vi "Odour_stim_valve_waveforms.vi"(1 "Odour bottles":T1(array[cluster])=[[{"Mixture components"=[{"Name"="MINERAL OIL", "CID"=0, "Volatility"=0.0}], "Name"="B1 (Bl)", "VPs"="0.0E+0", "Proportion"=[{"Numeric"=100.0}], "Selected"=FALSE, "Counter"=TRUE}, {"Mixture components"=[{"Name"="Methyl benzoate", "CID"=8103, "Volatility"=0.38}, {"Name"="Menthone", "CID"=8063, "Volatility"=0.28}], "Name"="B3 (ME2)", "VPs"="3.3E-1 ± 21%", "Proportion"=[{"Numeric"=50.0}, {"Numeric"=50.0}], "Selected"=TRUE, "Counter"=FALSE}, {"Mixture components"=[{"Name"="Decanol", "CID"=460, "Volatility"=0.00851}], "Name"="B5 (C4f)", "VPs"="8.5E-3", "Proportion"=[{"Numeric"=100.0}], "Selected"=FALSE, "Counter"=FALSE}, {"Mixture components"=[{"Name"="Acetophenone", "CID"=8174, "Volatility"=0.45}, {"Name"="Fenchone", "CID"=8635, "Volatility"=0.82}], "Name"="B7 (ME1)", "VPs"="6.4E-1 ± 41%", "Proportion"=[{"Numeric"=50.0}, {"Numeric"=50.0}], "Selected"=FALSE, "Counter"=FALSE}], [{"Mixture components"=[{"Name"="MINERAL OIL", "CID"=0, "Volatility"=0.0}], "Name"="B2 (Bl)", "VPs"="0.0E+0", "Proportion"=[{"Numeric"=100.0}], "Selected"=FALSE, "Counter"=TRUE}, {"Mixture components"=[{"Name"="Octanol", "CID"=7439, "Volatility"=0.0794}], "Name"="B4 (C4cA)", "VPs"="7.9E-2", "Proportion"=[{"Numeric"=100.0}], "Selected"=FALSE, "Counter"=FALSE}, {"Mixture components"=[{"Name"="MINERAL OIL", "CID"=0, "Volatility"=0.0}], "Name"="B6 (Bl)", "VPs"="0.0E+0", "Proportion"=[{"Numeric"=100.0}], "Selected"=FALSE, "Counter"=FALSE}, {"Mixture components"=[{"Name"="Heptanoic acid ", "CID"=957, "Volatility"=0.0107}], "Name"="B8 (C3cA)", "VPs"="1.1E-2", "Proportion"=[{"Numeric"=100.0}], "Selected"=FALSE, "Counter"=FALSE}], [{"Mixture components"=[{"Name"="MINERAL OIL", "CID"=0, "Volatility"=0.0}], "Name"="B9 (Bl)", "VPs"="0.0E+0", "Proportion"=[{"Numeric"=100.0}], "Selected"=FALSE, "Counter"=TRUE}, {"Mixture components"=[{"Name"="Geranyl acetate", "CID"=6985, "Volatility"=0.03}, {"Name"="Dimethylacetophenone", "CID"=7144, "Volatility"=0.063}], "Name"="B11 (MW1)", "VPs"="4.6E-2 ± 50%", "Proportion"=[{"Numeric"=50.0}, {"Numeric"=50.0}], "Selected"=FALSE, "Counter"=FALSE}, {"Mixture components"=[{"Name"="Geraniol", "CID"=6405, "Volatility"=0.03}, {"Name"="Phenyl butanone", "CID"=7762, "Volatility"=0.1}], "Name"="B13 (MW2)", "VPs"="6.5E-2 ± 76%", "Proportion"=[{"Numeric"=50.0}, {"Numeric"=50.0}], "Selected"=FALSE, "Counter"=FALSE}, {"Mixture components"=[{"Name"="Methylheptanoic acid", "CID"=1032, "Volatility"=0.018}], "Name"="B15 (C3f)", "VPs"="1.8E-2", "Proportion"=[{"Numeric"=100.0}], "Selected"=FALSE, "Counter"=FALSE}], [{"Mixture components"=[{"Name"="MINERAL OIL", "CID"=0, "Volatility"=0.0}], "Name"="B10 (Bl)", "VPs"="0.0E+0", "Proportion"=[{"Numeric"=100.0}], "Selected"=FALSE, "Counter"=TRUE}, {"Mixture components"=[{"Name"="Valeric acid", "CID"=8025, "Volatility"=0.196}], "Name"="B12 (C3cB)", "VPs"="2.0E-1", "Proportion"=[{"Numeric"=100.0}], "Selected"=FALSE, "Counter"=FALSE}, {"Mixture components"=[{"Name"="Nonanol", "CID"=4133, "Volatility"=0.0227}], "Name"="B14 (C4cB)", "VPs"="2.3E-2", "Proportion"=[{"Numeric"=100.0}], "Selected"=FALSE, "Counter"=FALSE}, {"Mixture components"=[{"Name"="Hydroxacetophenone", "CID"=7462, "Volatility"=0.0856}], "Name"="B16 (Ol)", "VPs"="8.6E-2", "Proportion"=[{"Numeric"=100.0}], "Selected"=FALSE, "Counter"=FALSE}]], 2 "Olfactormeter parameters":T2={"Back valve ON delays"=[0.0, 0.0, 0.0, 0.0, 0.0, 0.0, 0.0, 0.0, 0.0, 0.0, 0.0, 0.0, 0.0, 0.0, 0.0, 0.0], "Back valve OFF delays"=[0.0, 0.0, 0.0, 0.0, 0.0, 0.0, 0.0, 0.0, 0.0, 0.0, 0.0, 0.0, 0.0, 0.0, 0.0, 0.0], "Step duration (ms)"=2.0, "TTL binary step duration (ms)"=1.0, "Sampling rate (Hz)"=20000.0, "Initial delay (ms)"=250.0, "Pulse duration (ms)"=250.0} {"Initial delay (ms)" format="%#_13g"}, 3 "Stimulus parameters":T3={"Name"="Proba", "Active bottles"=[3], "Concentrations"=[1.0], "Unit"=enum."ppm"}) -> (0 "waveform array":digitalwaveform[](array[waveform])=[{"t0"=timestamp(0 s since 1904-01-01), "dt"=5e-05, "Y"={"transitions"=[], "data"=array5001x1[5001 elements]}, "attributes"=variant("NI_LineNames"=variant(string "Front valve 1"))}, {"t0"=timestamp(0 s since 1904-01-01), "dt"=5e-05, "Y"={"transitions"=[], "data"=array10001x1[10001 elements]}, "attributes"=variant("NI_LineNames"=variant(string "Front valve 2"))}, {"t0"=timestamp(0 s since 1904-01-01), "dt"=5e-05, "Y"={"transitions"=[], "data"=array10001x1[10001 elements]}, "attributes"=variant("NI_LineNames"=variant(string "Front valve 3"))}, {"t0"=timestamp(0 s since 1904-01-01), "dt"=5e-05, "Y"={"transitions"=[], "data"=[]}, "attributes"=variant("NI_LineNames"=variant(string "Front valve 4"))}, {"t0"=timestamp(0 s since 1904-01-01), "dt"=5e-05, "Y"={"transitions"=[], "data"=array10001x1[10001 elements]}, "attributes"=variant("NI_LineNames"=variant(string "Front valve 5"))}, {"t0"=timestamp(0 s since 1904-01-01), "dt"=5e-05, "Y"={"transitions"=[], "data"=array10001x1[10001 elements]}, "attributes"=variant("NI_LineNames"=variant(string "Front valve 6"))}, {"t0"=timestamp(0 s since 1904-01-01), "dt"=5e-05, "Y"={"transitions"=[], "data"=array10001x1[10001 elements]}, "attributes"=variant("NI_LineNames"=variant(string "Front valve 7"))}, {"t0"=timestamp(0 s since 1904-01-01), "dt"=5e-05, "Y"={"transitions"=[], "data"=array10001x1[10001 elements]}, "attributes"=variant("NI_LineNames"=variant(string "Front valve 8"))}, {"t0"=timestamp(0 s since 1904-01-01), "dt"=5e-05, "Y"={"transitions"=[], "data"=array10001x1[10001 elements]}, "attributes"=variant("NI_LineNames"=variant(string "Front valve 9"))}, {"t0"=timestamp(0 s since 1904-01-01), "dt"=5e-05, "Y"={"transitions"=[], "data"=array10001x1[10001 elements]}, "attributes"=variant("NI_LineNames"=variant(string "Front valve 10"))}, {"t0"=timestamp(0 s since 1904-01-01), "dt"=5e-05, "Y"={"transitions"=[], "data"=array10001x1[10001 elements]}, "attributes"=variant("NI_LineNames"=variant(string "Front valve 11"))}, {"t0"=timestamp(0 s since 1904-01-01), "dt"=5e-05, "Y"={"transitions"=[], "data"=array10001x1[10001 elements]}, "attributes"=variant("NI_LineNames"=variant(string "Front valve 12"))}, {"t0"=timestamp(0 s since 1904-01-01), "dt"=5e-05, "Y"={"transitions"=[], "data"=array10001x1[10001 elements]}, "attributes"=variant("NI_LineNames"=variant(string "Front valve 13"))}, {"t0"=timestamp(0 s since 1904-01-01), "dt"=5e-05, "Y"={"transitions"=[], "data"=array10001x1[10001 elements]}, "attributes"=variant("NI_LineNames"=variant(string "Front valve 14"))}, {"t0"=timestamp(0 s since 1904-01-01), "dt"=5e-05, "Y"={"transitions"=[], "data"=array10001x1[10001 elements]}, "attributes"=variant("NI_LineNames"=variant(string "Front valve 15"))}, {"t0"=timestamp(0 s since 1904-01-01), "dt"=5e-05, "Y"={"transitions"=[], "data"=array10001x1[10001 elements]}, "attributes"=variant("NI_LineNames"=variant(string "Front valve 16"))}, {"t0"=timestamp(0 s since 1904-01-01), "dt"=5e-05, "Y"={"transitions"=[], "data"=[]}, "attributes"=variant("NI_LineNames"=variant(string "Back valve 1"))}, {"t0"=timestamp(0 s since 1904-01-01), "dt"=5e-05, "Y"={"transitions"=[], "data"=[]}, "attributes"=variant("NI_LineNames"=variant(string "Back valve 2"))}, {"t0"=timestamp(0 s since 1904-01-01), "dt"=5e-05, "Y"={"transitions"=[], "data"=[]}, "attributes"=variant("NI_LineNames"=variant(string "Back valve 3"))}, {"t0"=timestamp(0 s since 1904-01-01), "dt"=5e-05, "Y"={"transitions"=[], "data"=[]}, "attributes"=variant("NI_LineNames"=variant(string "Back valve 4"))}, {"t0"=timestamp(0 s since 1904-01-01), "dt"=5e-05, "Y"={"transitions"=[], "data"=[]}, "attributes"=variant("NI_LineNames"=variant(string "Back valve 5"))}, {"t0"=timestamp(0 s since 1904-01-01), "dt"=5e-05, "Y"={"transitions"=[], "data"=[]}, "attributes"=variant("NI_LineNames"=variant(string "Back valve 6"))}, {"t0"=timestamp(0 s since 1904-01-01), "dt"=5e-05, "Y"={"transitions"=[], "data"=[]}, "attributes"=variant("NI_LineNames"=variant(string "Back valve 7"))}, {"t0"=timestamp(0 s since 1904-01-01), "dt"=5e-05, "Y"={"transitions"=[], "data"=[]}, "attributes"=variant("NI_LineNames"=variant(string "Back valve 8"))}, {"t0"=timestamp(0 s since 1904-01-01), "dt"=5e-05, "Y"={"transitions"=[], "data"=[]}, "attributes"=variant("NI_LineNames"=variant(string "Back valve 9"))}, {"t0"=timestamp(0 s since 1904-01-01), "dt"=5e-05, "Y"={"transitions"=[], "data"=[]}, "attributes"=variant("NI_LineNames"=variant(string "Back valve 10"))}, {"t0"=timestamp(0 s since 1904-01-01), "dt"=5e-05, "Y"={"transitions"=[], "data"=[]}, "attributes"=variant("NI_LineNames"=variant(string "Back valve 11"))}, {"t0"=timestamp(0 s since 1904-01-01), "dt"=5e-05, "Y"={"transitions"=[], "data"=[]}, "attributes"=variant("NI_LineNames"=variant(string "Back valve 12"))}, {"t0"=timestamp(0 s since 1904-01-01), "dt"=5e-05, "Y"={"transitions"=[], "data"=[]}, "attributes"=variant("NI_LineNames"=variant(string "Back valve 13"))}, {"t0"=timestamp(0 s since 1904-01-01), "dt"=5e-05, "Y"={"transitions"=[], "data"=[]}, "attributes"=variant("NI_LineNames"=variant(string "Back valve 14"))}, {"t0"=timestamp(0 s since 1904-01-01), "dt"=5e-05, "Y"={"transitions"=[], "data"=[]}, "attributes"=variant("NI_LineNames"=variant(string "Back valve 15"))}, {"t0"=timestamp(0 s since 1904-01-01), "dt"=5e-05, "Y"={"transitions"=[], "data"=[]}, "attributes"=variant("NI_LineNames"=variant(string "Back valve 16"))}, {"t0"=timestamp(0 s since 1904-01-01), "dt"=5e-05, "Y"={"transitions"=[], "data"=[]}, "attributes"=variant("NI_LineNames"=variant(string "Odour TTL1"))}])   [LabVIEW 2016]
uses:
  <vilib>/Waveform/DWDTOps.llb/DWDT Append Digital Signals.vi
panel:
  out "Digital Waveform Graph":digitalwaveform(graph)={"t0"=timestamp(0 s since 1904-01-01), "dt"=5e-05, "Y"={"transitions"=array[10001 elements], "data"=array10001x15[150015 elements]}, "attributes"=variant("NI_LineNames"=variant(string "Odour TTL1,Back valve 16,Back valve 15,Back valve 14,Back valve 13,Back valve 12,Back valve 11,Back valve 10,Back valve 9,Back valve 8,Back valve 7,Back valve 6,Back valve 5,Back valve 4,Back valve 3,Back valve 2,Back valve 1,Front valve 16,Front valve 15,Front valve 14,Front valve 13,Front valve 12,Front valve 11,Front valve 10,Front valve 9,Front valve 8,Front valve 7,Front valve 6,Front valve 5,Front valve 4,Front valve 3,Front valve 2,Front valve 1"))}
  out "Duty cycle":dbl[](array[numeric])=[0.0012125984251968502]
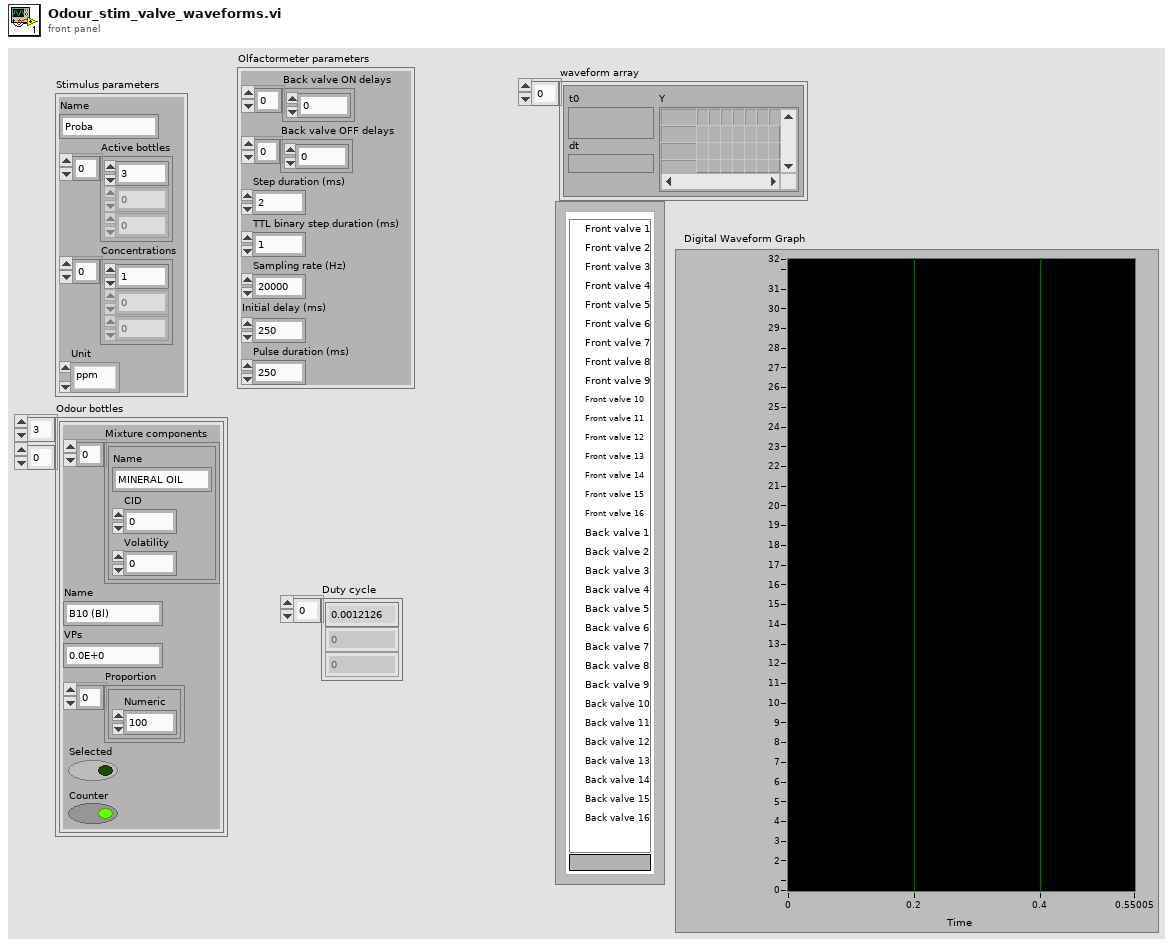
[diagram p1: front panel]
types:
  T1 = cluster{"Mixture components":cluster{"Name":string, "CID":i32, "Volatility":dbl}[], "Name":string, "VPs":string, "Proportion":cluster{"Numeric":dbl}[], "Selected":bool, "Counter":bool}[][]
  T2 = cluster{"Back valve ON delays":dbl[], "Back valve OFF delays":dbl[], "Step duration (ms)":dbl, "TTL binary step duration (ms)":dbl, "Sampling rate (Hz)":dbl, "Initial delay (ms)":dbl, "Pulse duration (ms)":dbl}
  T3 = cluster{"Name":string, "Active bottles":i32[], "Concentrations":dbl[], "Unit":enum16{"%", "ppm"}}
  T4 = cluster{"Initial phase":i32, "Back-valve pre-phase ":i32, "Main phase":i32, "Back-valve post-phase":i32, "Reset":i32, "Step":i32, "Total":i32, "ON delays":i32[], "OFF delays":i32[]}
  T5 = cluster{"Active bottles":i32[], "Counter bottles":i32[], "All counters":i32[]}
  T6 = enum16{"Inactive odour", "Active counter", "Inactive counter", "Active odour", "INVALID"}
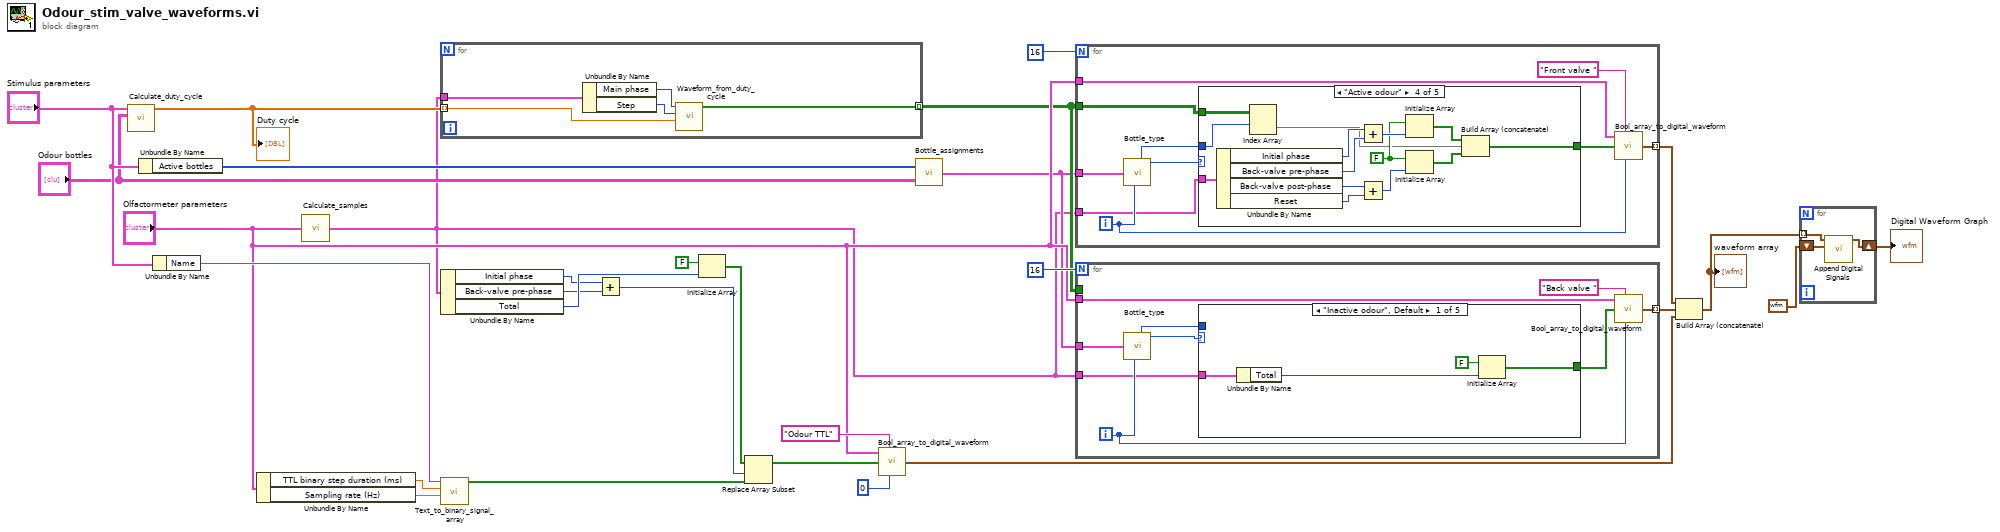
[diagram p0: block diagram]
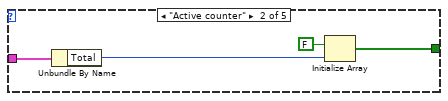
[diagram p2: hidden frame]
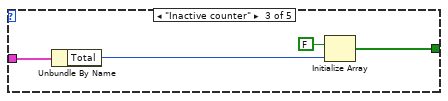
[diagram p3: hidden frame]
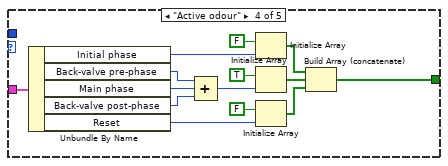
[diagram p4: hidden frame]
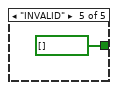
[diagram p5: hidden frame]
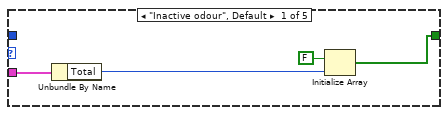
[diagram p6: hidden frame]
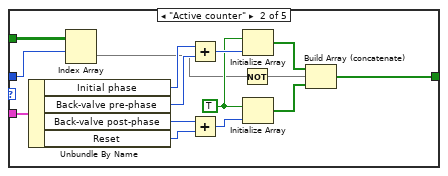
[diagram p7: hidden frame]
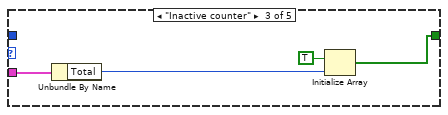
[diagram p8: hidden frame]
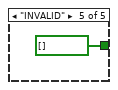
[diagram p9: hidden frame]
diagram:
  n1 = call "Calculate_duty_cycle.vi"("Odour bottles in"="Odour bottles", "Stimulus parameters"="Stimulus parameters") -> ("Duty cycle"=w27:dbl[])  [unwired: 9 in]
  "Duty cycle" <- w27
  n2 = Unbundle By Name("Stimulus parameters") -> ("Active bottles"=w24:i32[])
  n3 = Unbundle By Name("Stimulus parameters") -> ("Name"=w28:string)
  n4 = Unbundle By Name("Olfactormeter parameters") -> ("TTL binary step duration (ms)"=w29:dbl, "Sampling rate (Hz)"=w23:dbl)
  n5 = call "Calculate_samples.vi"("Olfactormeter parameters"="Olfactormeter parameters") -> ("Samples"=w8:T4)  [unwired: 4 in]
  n6 = for {
    tunnel: w27 -> [w34] mode=indexing
    tunnel: w8 -> [w32]
    tunnel: [w33] -> w11 mode=indexing
    n7 = Unbundle By Name(w32) -> ("Main phase"=w31:i32, "Step"=w30:i32)
    n8 = call "Waveform_from_duty_cycle.vi"("Duty cycle"=w34, "Step samples"=w30, "Total samples"=w31) -> ("odour waveform array"=w33:bool[])  [unwired: 8 in]
  }
  n9 = Unbundle By Name(w8) -> ("Initial phase"=w5:i32, "Back-valve pre-phase"=w4:i32, "Total"=w7:i32)
  n10 = call "Text_to_binary_signal_array.vi"("Sampling rate (Hz)"=w23, "TTL binary step duration (ms)"=w29, "Text"=w28) -> ("Signal array"=w2:bool[])  [unwired: 8 in]
  n11 = Add(x=w5, y=w4) -> (x+y=w3:i32)
  n12 = Initialize Array(FALSE, w7) -> (w6:bool[])
  n13 = Replace Array Subset(array=w6, new element=w2, index=w3) -> (w1:bool[])
  n14 = call "Bool_array_to_digital_waveform.vi"("Olfactormeter parameters"="Olfactormeter parameters", "Type"="Odour TTL" ("name"), "odour waveform array"=w1, "i"=0) -> ("digital waveform"=w12:digitalwaveform)  [unwired: 3 in]
  n15 = call "Bottle_assignments.vi"("Odour bottles"="Odour bottles", "Active bottles"=w24) -> ("Bottle assignments"=w10:T5)
  n16 = for {
    N: 16 -> [_]
    tunnel: w11 -> [w37]
    tunnel: w10 -> [w41]
    tunnel: "Olfactormeter parameters" -> [w44]
    tunnel: [w43] -> w16 mode=indexing
    tunnel: w8 -> [w38]
    i -> [w40]
    n17 = call "Bottle_type.vi"("Bottle assignments"=w41, "i"=w40) -> ("active bottle index"=w36:i32, "Bottle type"=w35:T6)  [unwired: 7 in]
    n18 = case shown="\"Active odour\"" w35 {
      tunnel: [w47 w51 w66 w69 bool[] []] -> w39
      tunnel: w38 -> [w46 w63 w65 w71 _]
      tunnel: w37 -> [_ w58 _ w72 _]
      tunnel: w36 -> [_ w49 _ w70 _]
      frame "Inactive odour", Default {
        n19 = Unbundle By Name(w46) -> ("Total"=w45:i32)
        n20 = Initialize Array(FALSE, w45) -> (w47:bool[])
      }
      frame "Active counter" {
        w53 = TRUE
        n21 = Unbundle By Name(w63) -> ("Initial phase"=w62:i32, "Back-valve pre-phase"=w61:i32, "Back-valve post-phase"=w56:i32, "Reset"=w55:i32)
        n22 = Index Array(array=w58, index (row)=w49) -> (element=w50:bool[])  [unwired: 1 in]
        n23 = Add(x=w62, y=w61) -> (x+y=w60:i32)
        n24 = Add(x=w56, y=w55) -> (x+y=w54:i32)
        n25 = Not(x=w50) -> (.not. x?=w57:bool[])
        n26 = Initialize Array(w53, w60) -> (w59:bool[])
        n27 = Initialize Array(w53, w54) -> (w52:bool[])
        n28 = Build Array (concatenate)(w59, w57, w52) -> (w51:bool[])
      }
      frame "Inactive counter" {
        n29 = Unbundle By Name(w65) -> ("Total"=w64:i32)
        n30 = Initialize Array(TRUE, w64) -> (w66:bool[])
      }
      frame "Active odour" {
        w74 = FALSE
        n31 = Unbundle By Name(w71) -> ("Initial phase"=w81:i32, "Back-valve pre-phase"=w80:i32, "Back-valve post-phase"=w77:i32, "Reset"=w76:i32)
        n32 = Index Array(array=w72, index (row)=w70) -> (element=w68:bool[])  [unwired: 1 in]
        n33 = Add(x=w81, y=w80) -> (x+y=w79:i32)
        n34 = Add(x=w77, y=w76) -> (x+y=w75:i32)
        n35 = Initialize Array(w74, w79) -> (w78:bool[])
        n36 = Initialize Array(w74, w75) -> (w73:bool[])
        n37 = Build Array (concatenate)(w78, w68, w73) -> (w69:bool[])
      }
      frame "INVALID" {
      }
    }
    n38 = call "Bool_array_to_digital_waveform.vi"("Olfactormeter parameters"=w44, "Type"="Front valve ", "odour waveform array"=w39, "i"=w40) -> ("digital waveform"=w43:digitalwaveform)  [unwired: 3 in]
  }
  n39 = for {
    N: 16 -> [_]
    tunnel: [w89] -> w22 mode=indexing
    tunnel: "Olfactormeter parameters" -> [w91]
    tunnel: w11 -> [_]
    tunnel: w10 -> [w87]
    tunnel: w8 -> [w84]
    i -> [w88]
    n40 = call "Bottle_type.vi"("Bottle assignments"=w87, "i"=w88) -> ("active bottle index"=w85:i32, "Bottle type"=w86:T6)  [unwired: 7 in]
    n41 = case shown="\"Inactive odour\", Default" w86 {
      tunnel: w84 -> [w94 w97 w102 w117 _]
      tunnel: w85 -> [_ _ _ _ _]
      tunnel: [w92 w96 w100 w104 bool[] []] -> w83
      frame "Inactive odour", Default {
        n42 = Unbundle By Name(w94) -> ("Total"=w93:i32)
        n43 = Initialize Array(FALSE, w93) -> (w92:bool[])
      }
      frame "Active counter" {
        n44 = Unbundle By Name(w97) -> ("Total"=w99:i32)
        n45 = Initialize Array(FALSE, w99) -> (w96:bool[])
      }
      frame "Inactive counter" {
        n46 = Unbundle By Name(w102) -> ("Total"=w101:i32)
        n47 = Initialize Array(FALSE, w101) -> (w100:bool[])
      }
      frame "Active odour" {
        n48 = Unbundle By Name(w117) -> ("Initial phase"=w115:i32, "Back-valve pre-phase"=w113:i32, "Main phase"=w112:i32, "Back-valve post-phase"=w111:i32, "Reset"=w106:i32)
        n49 = Compound Arithmetic op=ADD(w113, w112, w111) -> (w110:i32)
        n50 = Initialize Array(FALSE, w115) -> (w109:bool[])
        n51 = Initialize Array(TRUE, w110) -> (w108:bool[])
        n52 = Initialize Array(FALSE, w106) -> (w105:bool[])
        n53 = Build Array (concatenate)(w109, w108, w105) -> (w104:bool[])
      }
      frame "INVALID" {
      }
    }
    n54 = call "Bool_array_to_digital_waveform.vi"("Olfactormeter parameters"=w91, "Type"="Back valve ", "odour waveform array"=w83, "i"=w88) -> ("digital waveform"=w89:digitalwaveform)  [unwired: 3 in]
  }
  n55 = Build Array (concatenate)(w16, w22, w12) -> (w19:digitalwaveform[])
  "waveform array" <- w19
  n56 = for {
    shift-right: [w121] -> w18
    shift-left: digitalwaveform {"t0"=timestamp(0 s since 1904-01-01), "dt"=0.0, "Y"={"transitions"=[], "data"=[]}} ("waveform out") -> [w120]
    tunnel: w19 -> [w119] mode=indexing
    n57 = call-poly <vilib>:"Append Digital Signals.vi"("digital waveform (low bits)"=w120, "digital waveform (high bits)"=w119) -> ("digital waveform out"=w121:digitalwaveform)  [unwired: 8 in, 1 out]
  }
  "Digital Waveform Graph" <- w18
